vi "Configure Units.vi"(7 "Channel (0: Channel A)":u16(ring) items=["Channel A", "Channel B"], 8 "error in (no error)":errorcluster, 10 "Unit (mbar)":u16(ring) items=["mbar", "bar", "Pa", "hPa", "kPa", "mPa", "mmHg@0°C", "cmHg@0°C", "mHg@0°C", "inHg@0°C", "kg/cm2", "kg/m2", "mmH2O@4°C", "cmH2O@4°C", "mH2O@4°C", "mmH2O@20°C", "cmH2O@20°C", "mH2O@20°C", "torr", "atm", "psi", "lb/ft2", "inH2O@4°C", "inH2O@20°C", "inH2O@60°F", "ftH2O@4°C", "ftH2O@20°C", "ftH2O@60°F", "UserUnit1", "UserUnit2", "UserUnit3", "UserUnit4"], 11 "BH Druck PACE Series in":refnum<class "BH Druck PACE Series.lvclass">) -> (0 "error out":errorcluster, 3 "BH Druck PACE Series out":refnum<class "BH Druck PACE Series.lvclass">)   [LabVIEW 2022 SP3, in "BH Druck PACE Series.lvclass"]
uses:
  BH Druck PACE Series.lvclass
  BH Druck PACE Series.lvclass/BH Druck PACE Series.ctl
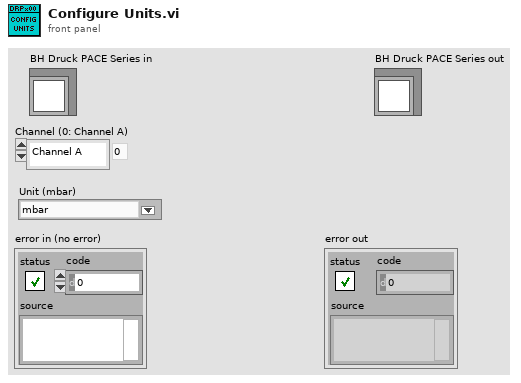
[diagram p1: front panel]
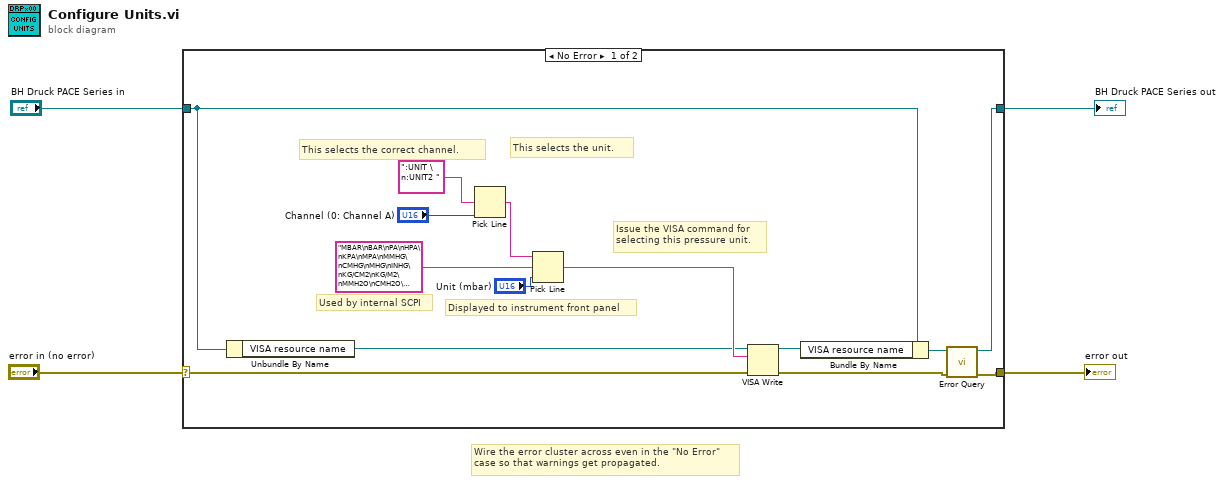
[diagram p0: block diagram]
diagram:
  # "Wire the error cluster across even in the \"No Error\"\ncase so that warnings get propagated."
  n1 = case shown="No Error" "error in (no error)" {
    selector: "error in (no error)" -> [w12 w20]
    tunnel: [w5 w20] -> w3
    tunnel: [w6 w19] -> w1
    tunnel: "BH Druck PACE Series in" -> [w10 w19]
    frame No Error {
      # "Displayed to instrument front panel"
      # "Used by internal SCPI"
      # "This selects the unit."
      # "This selects the correct channel."
      # "Issue the VISA command for\nselecting this pressure unit."
      n2 = Unbundle By Name(w10) -> ("VISA resource name"=w11:refnum<visa-resource-name>)
      n3 = Pick Line(multi-line string=":UNIT \n:UNIT2 ", line index="Channel (0: Channel A)") -> (output string=w13:string)  [unwired: 1 in]
      n4 = Pick Line(string ("")=w13, multi-line string="MBAR\nBAR\nPA\nHPA\nKPA\nMPA\nMMHG\nCMHG\nMHG\nINHG\nKG/CM2\nKG/M2\nMMH2O\nCMH2O\nMH2O\nMMH2O20\nCMH2O20\nMH2O20\nTORR\nATM\nPSI\nLB/FT2\nINH2O4\nINH2O\nINH2O60\nFTH2O4\nFTH2O\nFTH2O60\nUSER1\nUSER2\nUSER3\nUSER4", line index="Unit (mbar)") -> (output string=w14:string)
      n5 = VISA Write(VISA resource name=w11, write buffer=w14, error in (no error)=w12) -> (VISA resource name out=w9:refnum<visa-resource-name>, error out=w8:errorcluster)  [unwired: 1 out]
      n6 = Bundle By Name(cluster=w10, "VISA resource name"=w9) -> (w7:refnum<class "BH Druck PACE Series.lvclass">)
      n7 = call-dynamic "Error Query.vi"("error in (no error)"=w8, "BH Druck PACE Series in"=w7) -> ("error out"=w5:errorcluster, "BH Druck PACE Series out"=w6:refnum<class "BH Druck PACE Series.lvclass">)  [unwired: 8 in]
    }
    frame Error {
    }
  }
  "error out" <- w3
  "BH Druck PACE Series out" <- w1
